vi "add_vectors.vi"(0 "vector_weviate in":refnum<class "vector_weviate.lvclass">, 5 "colection_name":string, 7 "vectors":T1[](array[typedef]), 11 "error in (no error)":errorcluster) -> (4 "vector_weviate out":refnum<class "vector_weviate.lvclass">, 15 "error out":errorcluster)   [LabVIEW 2020, in "vector_weviate.lvclass"]
uses:
  vector_weviate.lvclass
  abstract_vector_base/vector.ctl
  vector_weviate.lvclass/vector_weviate.ctl
  <vilib>/httpClient/POSTBuffer.vi
  <vilib>/httpClient/LabVIEWHTTPClient.lvlib
  abstract_vector_base/abstract_vector_base.lvclass
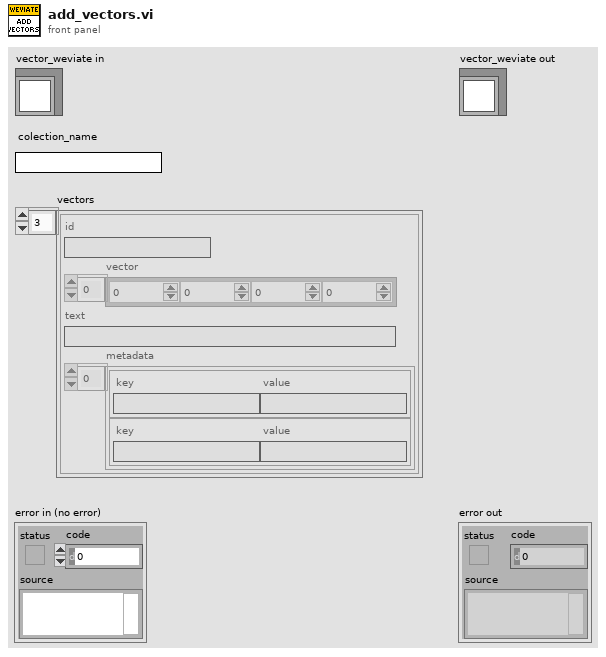
[diagram p1: front panel]
types:
  T1 = typedef "abstract_vector_base.lvclass/vector.ctl" = cluster{"id":string, "vector":dbl[], "text":string, "metadata":cluster{"key":string, "value":string}[]}
  T2 = cluster{"Class":string, "id":string, "properties":cluster{"text":string}, "vector":dbl[]}
  T3 = cluster{"Objects":cluster{"Class":string, "id":string, "properties":cluster{"text":string}, "vector":dbl[]}[]}
  T4 = typedef "LabVIEWHTTPClient.lvlib/ClientHandle.ctl" = refnum<k1>
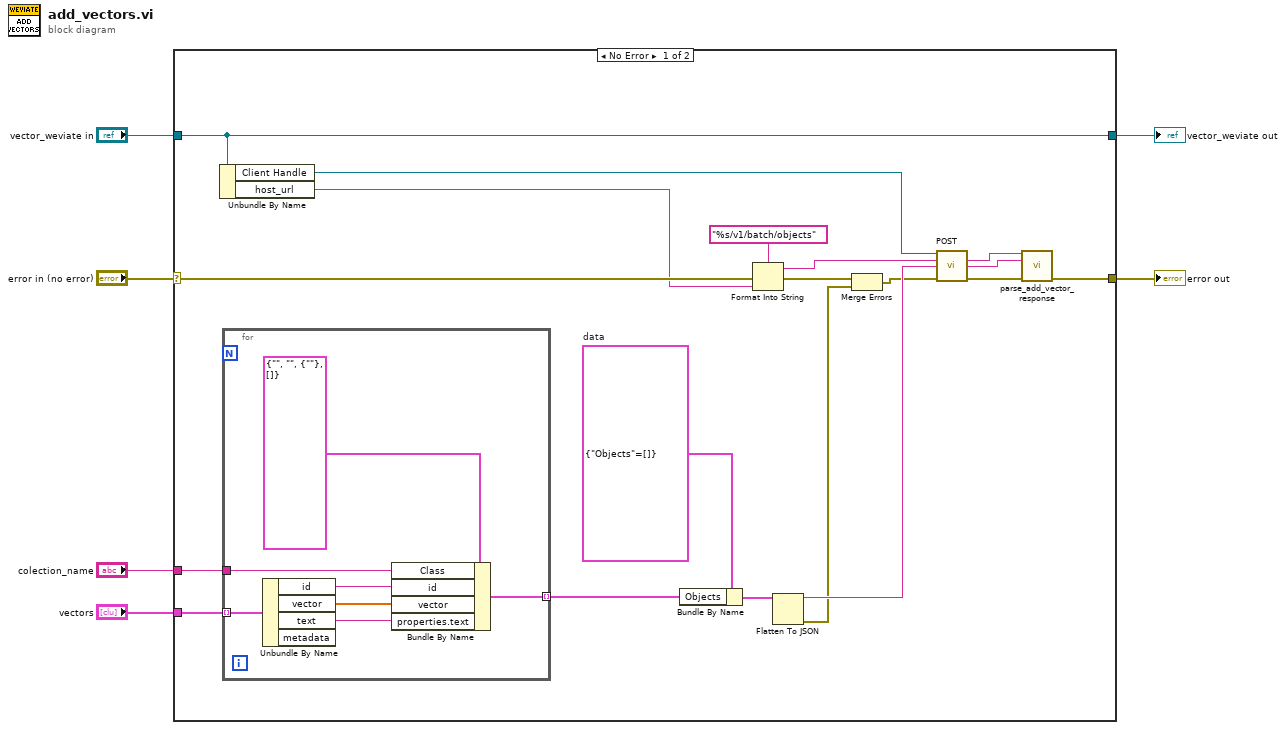
[diagram p0: block diagram]
diagram:
  n1 = case shown="No Error" "error in (no error)" {
    selector: "error in (no error)" -> [w20 w33]
    tunnel: "vectors" -> [w25 _]
    tunnel: "colection_name" -> [w21 _]
    tunnel: "vector_weviate in" -> [w11 w34]
    tunnel: [w11 w34] -> w2
    tunnel: [w7 w33] -> w1
    frame No Error {
      w22 = T3 {"Objects"=[]}  # data
      n2 = Unbundle By Name(w11) -> ("Client Handle"=w17:T4, "host_url"=w19:string)
      n3 = for {
        tunnel: w25 -> [w32] mode=indexing
        tunnel: [w27] -> w24 mode=indexing
        tunnel: w21 -> [w26]
        n4 = Unbundle By Name(w32) -> ("id"=w30:string, "vector"=w29:dbl[], "text"=w28:string)  [unwired: 1 out]
        n5 = Bundle By Name(cluster=T2 {"Class"="", "id"="", "properties"={"text"=""}, "vector"=[]}, "Class"=w26, "id"=w30, "vector"=w29, "properties.text"=w28) -> (w27:T2)
      }
      n6 = Bundle By Name(cluster=w22, "Objects"=w24) -> (w23:T3)
      n7 = Format Into String(format string="%s/v1/batch/objects", error in=w20, w19) -> (resulting string=w16:string, error out=w14:errorcluster)  [unwired: 1 in]
      n8 = Flatten To JSON(anything=w23) -> (JSON string=w15:string, 11:w13:errorcluster)  [unwired: 2 in]
      n9 = Merge Errors(w14, w13) -> (w12:errorcluster)
      n10 = call-poly <vilib>:"POST.vi"("client handle"=w17, "url"=w16, "buffer"=w15, "error in (no error)"=w12) -> ("headers"=w9:string, "body"=w8:string, "error out"=w10:errorcluster)  [unwired: 8 in, 1 out]
      n11 = call "parse_add_vector_response.vi"("headers"=w9, "body"=w8, "error in (no error)"=w10) -> ("error out"=w7:errorcluster)  [unwired: 12 in]
    }
    frame Error {
    }
  }
  "error out" <- w1
  "vector_weviate out" <- w2
